vi "poly_notify_boolean_notifier_notifier.vi"(2 "notifier":T1) -> (7 "notified?":bool)   [LabVIEW 2015]
uses:
  cores/boolean_notifier.ctl
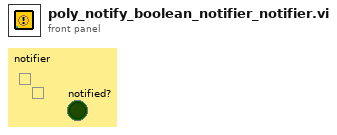
[diagram p1: front panel]
types:
  T1 = typedef "boolean_notifier.ctl" = refnum<queue>
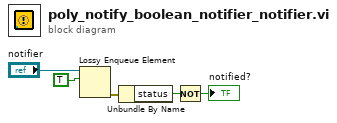
[diagram p0: block diagram]
diagram:
  n1 = Lossy Enqueue Element(queue="notifier", element=TRUE) -> (error out=w1:errorcluster)  [unwired: 1 in, 3 out]
  n2 = Unbundle By Name(w1) -> ("status"=w5:bool)
  n3 = Not(x=w5) -> (.not. x?=→"notified?":bool)
